vi "Validate Configuration.vi"(8 "error in":errorcluster, 11 "IValidateConfiguration in":refnum<class "PCAN Base Strategy.lvclass">) -> (0 "error out":errorcluster, 3 "IValidateConfiguration out":refnum<class "PCAN Base Strategy.lvclass">)   [LabVIEW 2024, in "PCAN Base Strategy.lvclass"]
uses:
  PCAN Base Strategy.lvclass
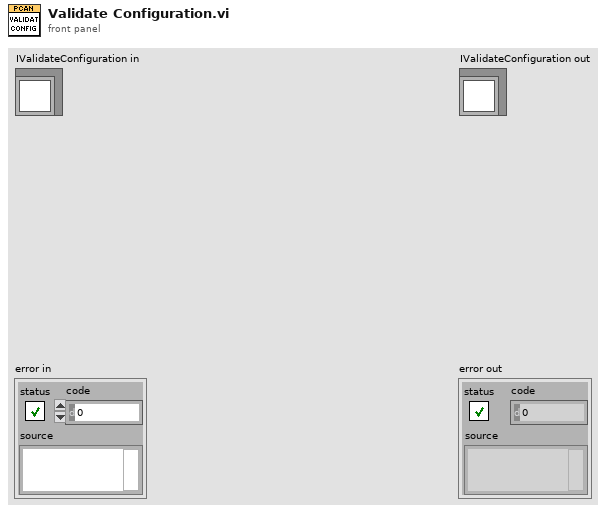
[diagram p1: front panel]
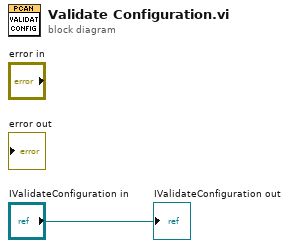
[diagram p0: block diagram]
diagram:
  "IValidateConfiguration out" <- "IValidateConfiguration in"
